vi "Get Class from TSM Context.vi"(0 "TSM Context":T1) -> (4 "Global Memory Class":refnum<class "TSM Context Data Access.lvclass">)   [LabVIEW 2019, in "TSM Context Data Access.lvclass"]
uses:
  TSM Context Data Access.lvclass
  <vilib>/NI_TestStand_SemiconductorModule/NI_TestStand_Semiconductor_Module.lvlibp/PinMap/General/SemiconductorModuleContext.ctl
  TSM Context Data Access.lvclass/TSM Context Data Access.ctl
  <vilib>/NI_TestStand_SemiconductorModule/NI_TestStand_Semiconductor_Module.lvlibp
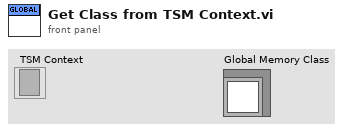
[diagram p1: front panel]
types:
  T1 = typedef "NI_TestStand_Semiconductor_Module.lvlibp/SemiconductorModuleContext.ctl" = refnum<k7>
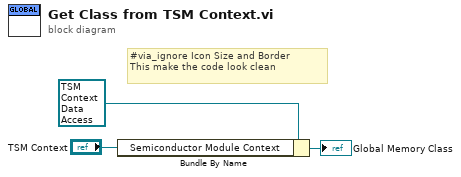
[diagram p0: block diagram]
diagram:
  # "#via_ignore Icon Size and Border\nThis make the code look clean"
  n1 = Bundle By Name(cluster=refnum<class "TSM Context Data Access.lvclass"> refnum ("TSM Context Global Access.lvclass"), "Semiconductor Module Context"="TSM Context") -> (→"Global Memory Class":refnum<class "TSM Context Data Access.lvclass">)
